vi "Graphics-LTRB to WHCM.vi"(7 "LTRB":T1) -> (0 "Middle":i16, 2 "Center":i16, 3 "Height":i16, 5 "Width":i16)   [LabVIEW 2020]
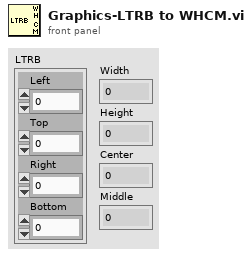
[diagram p1: front panel]
types:
  T1 = cluster{"Left":i16, "Top":i16, "Right":i16, "Bottom":i16}
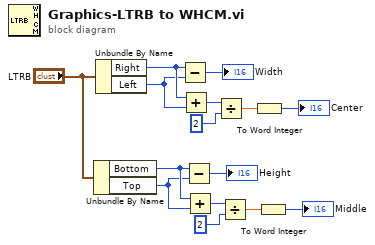
[diagram p0: block diagram]
diagram:
  n1 = Unbundle By Name("LTRB") -> ("Bottom"=w8:i16, "Top"=w7:i16)
  n2 = Unbundle By Name("LTRB") -> ("Right"=w15:i16, "Left"=w14:i16)
  n3 = Subtract(x=w15, y=w14) -> (x-y=→"Width":i16)
  n4 = Add(x=w15, y=w14) -> (x+y=w13:i16)
  n5 = Subtract(x=w8, y=w7) -> (x-y=→"Height":i16)
  n6 = Add(x=w8, y=w7) -> (x+y=w6:i16)
  n7 = Divide(x=w13, y=2) -> (x/y=w11:dbl)
  n8 = Divide(x=w6, y=2) -> (x/y=w4:dbl)
  n9 = To Word Integer(number=w11) -> (16bit integer=→"Center":i16)
  n10 = To Word Integer(number=w4) -> (16bit integer=→"Middle":i16)
